vi "Get inClosed.vi"(8 "error in (no error)":errorcluster, 11 "AbstractDstarNode in":refnum<class "NI_Robotics_AbstractDstarNode.lvclass">) -> (0 "error out":errorcluster, 2 "inClosed":i32, 3 "AbstractDstarNode out":refnum<class "NI_Robotics_AbstractDstarNode.lvclass">)   [LabVIEW 2017, in "NI_Robotics_AbstractDstarNode.lvclass"]
uses:
  <vilib>/robotics/Navigation/shared/MapNode/AbstractDstarNode/NI_Robotics_AbstractDstarNode.lvclass
  <vilib>/robotics/Navigation/shared/MapNode/AbstractDstarNode/NI_Robotics_AbstractDstarNode.lvclass/NI_Robotics_AbstractDstarNode.ctl
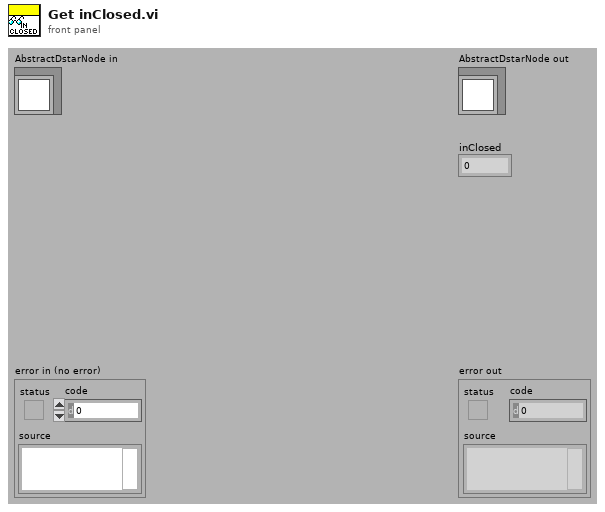
[diagram p1: front panel]
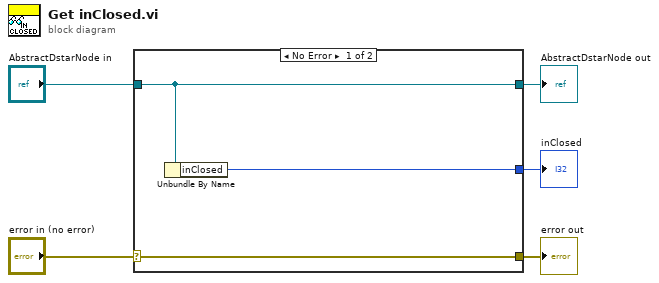
[diagram p0: block diagram]
diagram:
  n1 = case shown="No Error" "error in (no error)" {
    selector: "error in (no error)" -> [w8 w9]
    tunnel: [w8 w9] -> w4
    tunnel: [w7 w10] -> w2
    tunnel: "AbstractDstarNode in" -> [w7 w10]
    tunnel: [w6 _] -> w1
    frame No Error {
      n2 = Unbundle By Name(w7) -> ("inClosed"=w6:i32)
    }
    frame Error {
    }
  }
  "error out" <- w4
  "AbstractDstarNode out" <- w2
  "inClosed" <- w1
